vi "Enable_Disable Motor.vi"(8 "error in (no error)":errorcluster, 9 "enable/disable":bool, 10 "Index":i32, 11 "Motions in":refnum<class "Motions.lvclass">) -> (0 "error out":errorcluster, 3 "Motions out":refnum<class "Motions.lvclass">)   [LabVIEW 2016, in "Hardware.lvlib" / "Motions.lvlib" / "Motions.lvclass"]
uses:
  <userlib>/Common Components/Hardware/Abstract System/Motions/Motions/Motions.lvclass
  <userlib>/Common Components/Hardware/Abstract System/Motions/Motions/Motions.lvclass/Motions.ctl
  <userlib>/Common Components/Hardware/Motor/Motor/Motor.lvclass
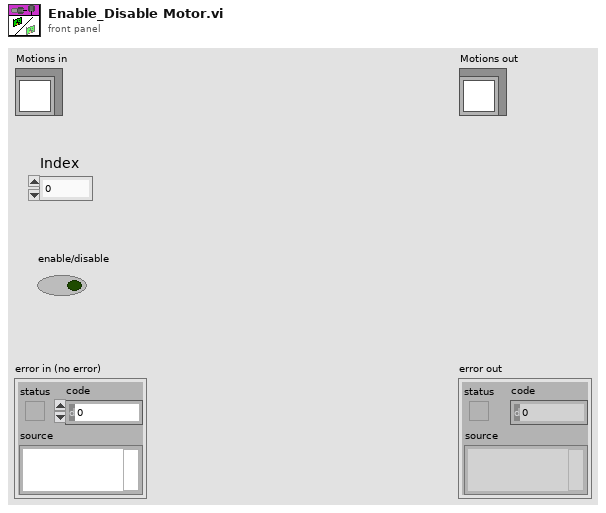
[diagram p1: front panel]
types:
  T1 = typedef "Hardware.lvlib/Motions.lvlib/Motions.lvclass/Motor States.ctl" = cluster{"Connected":bool, "Enabled":bool, "Moving Status":bool, "Soft Moving Status":bool, "Current Pos":dbl, "Target Pos":dbl, "Moving Dir (-1, 0, 1)":i32, "Error Status":bool, "Hard Limit+":bool, "Hard Limit-":bool, "Soft Limit+":bool, "Soft Limit-":bool, "History Dst Stack":refnum<queue>, "Motion Status":bool, "Motion TriggerAction Obj":refnum<class "TriggerAction Q.lvclass">}
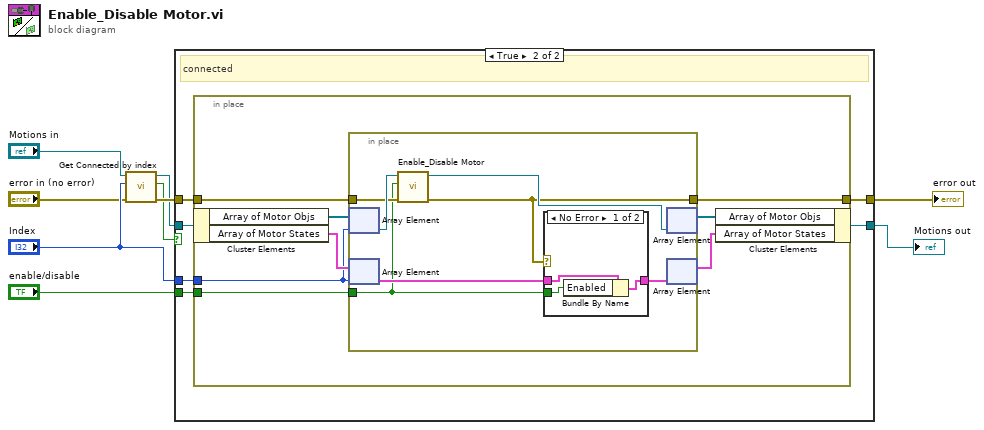
[diagram p0: block diagram]
diagram:
  n1 = call <userlib>:"Get Connected by index.vi"("error in (no error)"="error in (no error)", "index"="Index", "Motions in"="Motions in") -> ("error out"=w9:errorcluster, "Connected"=w7:bool, "Motions out"=w8:refnum<class "Motions.lvclass">)  [unwired: 6 in]
  n2 = case shown="True" w7 {
    tunnel: [w10 w17] -> w3
    tunnel: [w11 w16] -> w1
    tunnel: w9 -> [w11 w15]
    tunnel: w8 -> [w10 w14]
    tunnel: "Index" -> [_ w13]
    tunnel: "enable/disable" -> [_ w12]
    frame False {
    }
    frame True {
      # "connected"
      n3 = in-place {
        in-place-border: w13 -> [w19]
        in-place-border: w15 -> [w23]
        in-place-border: [w22] -> w16
        in-place-border: w12 -> [w21]
        n4 = in-place-cluster #1(w14) -> ("Array of Motor Objs"=w25:refnum<class "Motor.lvclass">[], "Array of Motor States"=w20:T1[])
        n5 = in-place {
          in-place-border: w23 -> [w30]
          in-place-border: [w26] -> w22
          in-place-border: w21 -> [w27]
          n6 = in-place-array #2(w25, w19) -> (w32:refnum<class "Motor.lvclass">)
          n7 = in-place-array #3(w20, w19) -> (w29:T1)
          n8 = call-dynamic "Enable_Disable Motor.vi"("error in (no error)"=w30, "enable/disable"=w27, "Motor in"=w32) -> ("error out"=w26:errorcluster, "Motor out"=w31:refnum<class "Motor.lvclass">)  [unwired: 7 in]
          n9 = case shown="No Error" w26 {
            tunnel: w29 -> [w35 w36]
            tunnel: [w34 w36] -> w28
            tunnel: w27 -> [w33 _]
            frame No Error {
              n10 = Bundle By Name(cluster=w35, "Enabled"=w33) -> (w34:T1)
            }
            frame Error {
            }
          }
          n11 = in-place-array #2(w31) -> (w24:refnum<class "Motor.lvclass">[])  [unwired: 1 out]
          n12 = in-place-array #3(w28) -> (w18:T1[])  [unwired: 1 out]
        }
        n13 = in-place-cluster #1("Array of Motor Objs"=w24, "Array of Motor States"=w18) -> (w17:refnum<class "Motions.lvclass">)
      }
    }
  }
  "error out" <- w1
  "Motions out" <- w3
